vi "No Error.vi"() -> ()   [LabVIEW 2017, in "Assertion.Tests.lvlib" / "Error Message Contains String.lvlib"]
uses:
  Error Message Contains String.lvlib
  a9cd2165-557e-43d9-abd3-def871d88858.vi
  Constraint/IsEqual/Create.vi
  Constraint/IsEqual/IsEqual.lvclass
  Assertion/Assertion.lvlib
  Assertion.Tests.lvlib
panel:
  out "error out":errorcluster
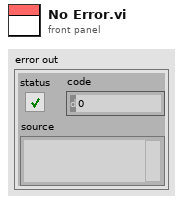
[diagram p1: front panel]
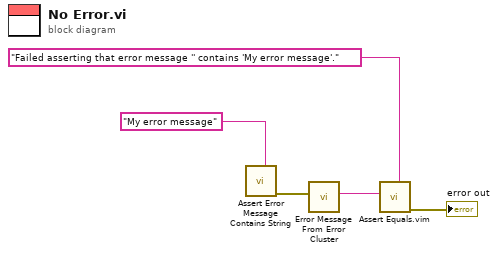
[diagram p0: block diagram]
diagram:
  n1 = call "Assert Error Message Contains String.vi"("Expected"="My error message") -> ("error out"=w2:errorcluster)  [unwired: 10 in]
  n2 = call "Error Message From Error Cluster.vi"("Error"=w2) -> ("Error Message"=w4:string)  [unwired: 10 in]
  n3 = call "Assert Equals.vim"("Expected"="Failed asserting that error message '' contains 'My error message'." ("Needle"), "Actual"=w4) -> ("error out"=→"error out":errorcluster)  [unwired: 9 in]
